vi "BlueSerialProviderGlobal.vi"() -> ()   [LabVIEW 2019, in "BlueSerializationScripts.lvlib"]
uses:
  BlueSerializationScripts.lvlib
panel:
  in  "SerializableData_v1.ctl":string="SerializableData_v1.ctl"
  in  "Mutate_v1_to_v2.vi":string="Mutate_v1_to_v2.vi"
  in  "ScriptedCaseStructure":string="ScriptedCaseStructure"
  in  "GetVersionSerializableData.vi":string="GetVersionSerializableData.vi"
  in  "Mutations":string="Mutations"
  in  "Mutate_Template.vi":string="Mutate_Template.vi"
  in  "HandleVersionMutation.vi":string="HandleVersionMutation.vi"
  in  "SetSerializableData.vi":string="SetSerializableData.vi"
  in  "SerializableData.ctl":string="SerializableData.ctl"
  in  "GetSerializableData.vi":string="GetSerializableData.vi"
  in  "SerializableData":string="SerializableData"
  in  "BlueSerialization":string="BlueSerialization"
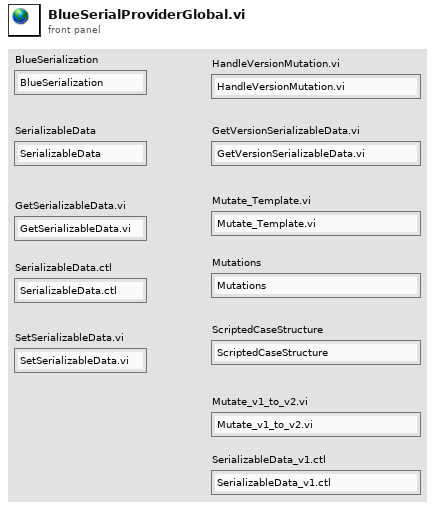
[diagram p1: front panel]
diagram:
